vi "Set Enable State on Multiple Controls.vi"(10 "Enable?":bool caption="启用？", 11 "Array of Ctrl Refs":refnum<vi>[](array[refnum]) caption="控件引用数组") -> ()   [LabVIEW 2013]
doc: "将输入数组中所有控件的值设置为“启用状态”。"
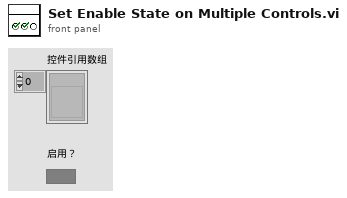
[diagram p1: front panel]
types:
  T1 = enum8{"Enabled", "Disabled", "Disabled and Grayed Out"}
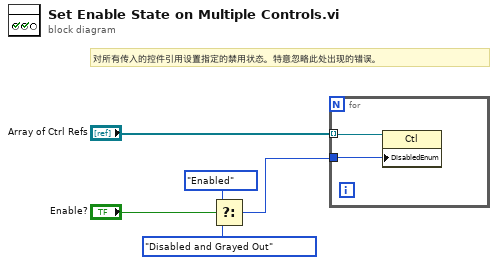
[diagram p0: block diagram]
diagram:
  # "对所有传入的控件引用设置指定的禁用状态。特意忽略此处出现的错误。"
  n1 = Select(t=T1."Enabled" ("Disabled"), s="Enable?", f=T1."Disabled and Grayed Out" ("Disabled")) -> (s? t:f=w4:T1)
  n2 = for {
    tunnel: "Array of Ctrl Refs" -> [w7] mode=indexing
    tunnel: w4 -> [w6]
    n3 = property class="Ctl"(reference=w7, "DisabledEnum"=w6) -> ()  [unwired: 1 in, 2 out]
  }
